vi "Cleanup.vi"(8 "error in (no error)":errorcluster, 11 "Vecto in":refnum<class "Vecto.lvclass">) -> (0 "error out":errorcluster)   [LabVIEW 2020, in "Vecto.lvlib" / "Vecto.lvclass"]
uses:
  Vecto.lvclass
  Vecto.lvclass/Vecto.ctl
  lv-http-server/HTTP Server/Server/Server.lvclass
  VectoService/VectoInfo.lvclass
  InfoService/NodeStatus.lvclass
  SequenceCountService/SequenceCountService.lvclass
  RemoteDataService/RemoteDataService.lvclass
  ChannelService/ChannelService.lvclass
  TCPMessaging/TCPMessaging.lvclass
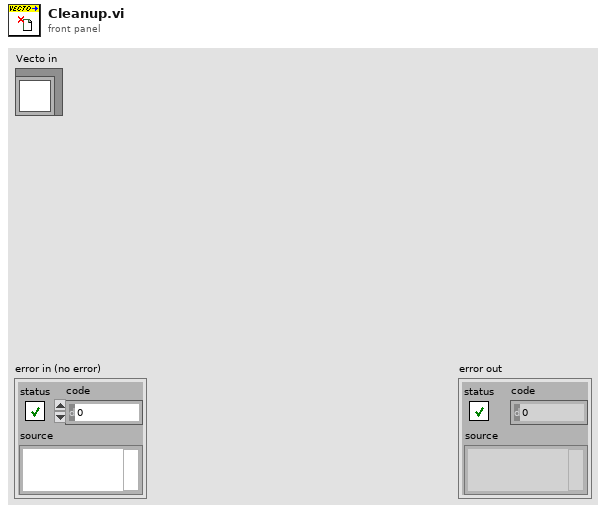
[diagram p1: front panel]
types:
  T1 = typedef "Vecto.lvlib/Vecto.lvclass/Local Services.ctl" = cluster{"InfoService":refnum<class "NodeStatus.lvclass">, "VectoService":refnum<class "VectoInfo.lvclass">, "ChannelService":refnum<class "ChannelService.lvclass">, "EventLogging":refnum<class "EventLoggingService.lvclass">}
  T2 = typedef "Vecto.lvlib/Vecto.lvclass/Remote Services.ctl" = cluster{"SequenceCountService":refnum<class "SequenceCountService.lvclass">, "RemoteDataService":refnum<class "RemoteDataService.lvclass">, "TCPMessaging":refnum<class "TCPMessaging.lvclass">}
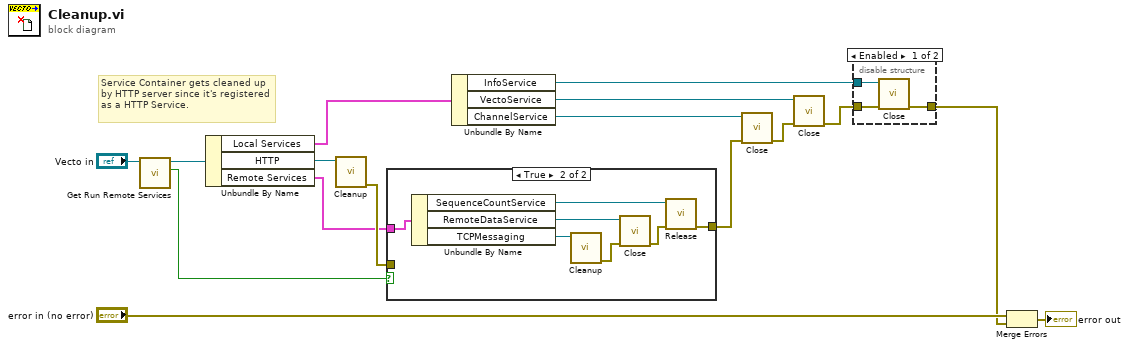
[diagram p0: block diagram]
diagram:
  # "Service Container gets cleaned up by HTTP server since it's registered as a HTTP Service."
  n1 = call "Get Run Remote Services.vi"("Vecto in"="Vecto in") -> ("Run Remote Services"=w7:bool, "Vecto out"=w8:refnum<class "Vecto.lvclass">)  [unwired: 8 in, 1 out]
  n2 = Unbundle By Name(w8) -> ("Local Services"=w14:T1, "HTTP"=w15:refnum<class "Server.lvclass">, "Remote Services"=w5:T2)
  n3 = call "Cleanup.vi"("Server in"=w15) -> ("error out"=w6:errorcluster)  [unwired: 10 in]
  n4 = case shown="True" w7 {
    tunnel: w6 -> [w17 _]
    tunnel: w5 -> [_ w24]
    tunnel: [w17 w22] -> w1
    frame False {
    }
    frame True {
      n5 = Unbundle By Name(w24) -> ("SequenceCountService"=w23:refnum<class "SequenceCountService.lvclass">, "RemoteDataService"=w21:refnum<class "RemoteDataService.lvclass">, "TCPMessaging"=w20:refnum<class "TCPMessaging.lvclass">)
      n6 = call "Cleanup.vi"("TCPMessaging in"=w20) -> ("error out"=w19:errorcluster)  [unwired: 10 in]
      n7 = call "Close.vi"("error in (no error)"=w19, "RemoteDataService in"=w21) -> ("error out"=w18:errorcluster)  [unwired: 9 in]
      n8 = call "Release.vi"("error in (no error)"=w18, "SequenceCountService in"=w23) -> ("error out"=w22:errorcluster)  [unwired: 9 in]
    }
  }
  n9 = Unbundle By Name(w14) -> ("InfoService"=w12:refnum<class "NodeStatus.lvclass">, "VectoService"=w13:refnum<class "VectoInfo.lvclass">, "ChannelService"=w3:refnum<class "ChannelService.lvclass">)
  n10 = call "Close.vi"("error in (no error)"=w1, "ChannelService in"=w3) -> ("error out"=w2:errorcluster)  [unwired: 9 in]
  n11 = call "Close.vi"("error in (no error)"=w2, "VectoService in"=w13) -> ("error out"=w11:errorcluster)  [unwired: 9 in]
  n12 = disable-structure shown="Enabled" {
    disable-tunnel: w12 -> [w27 _]
    disable-tunnel: w11 -> [w26 w28]
    disable-tunnel: [w25 w28] -> w4
    frame Enabled {
      n13 = call "Close.vi"("error in (no error)"=w26, "InfoService in"=w27) -> ("error out"=w25:errorcluster)  [unwired: 9 in]
    }
    frame Disabled {
    }
  }
  n14 = Merge Errors("error in (no error)", w4) -> (→"error out":errorcluster)
